vi "Write QueueMessageRef.vi"(8 "error in (no error)":errorcluster, 10 "QueueMessageRef":refnum<queue>, 11 "MicronGRPC in":refnum<class "MicronGRPC.lvclass">) -> (0 "error out":errorcluster, 3 "MicronGRPC out":refnum<class "MicronGRPC.lvclass">)   [LabVIEW 2019, in "MicronGRPCGeneratedServer.lvlib" / "MicronGRPC.lvclass"]
uses:
  MicronGRPC.lvclass
  Base/Server/Message/MessageBase.lvclass
  MicronGRPC.lvclass/MicronGRPC.ctl
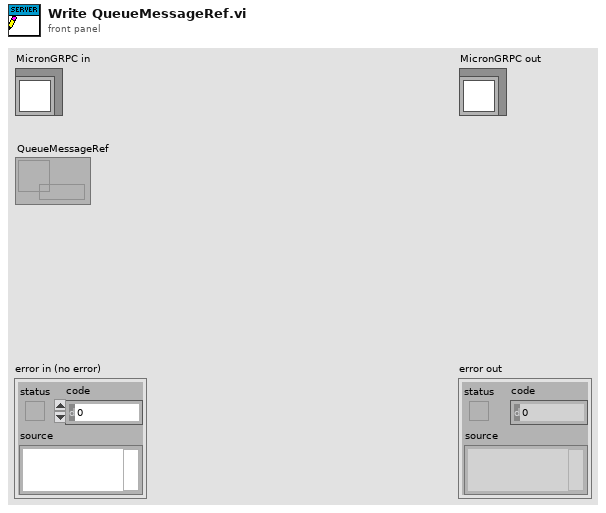
[diagram p1: front panel]
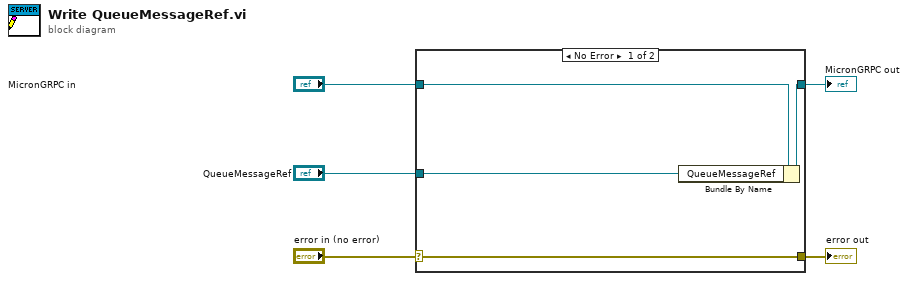
[diagram p0: block diagram]
diagram:
  n1 = case shown="No Error" "error in (no error)" {
    selector: "error in (no error)" -> [w9 w10]
    tunnel: [w9 w10] -> w4
    tunnel: [w7 w11] -> w2
    tunnel: "MicronGRPC in" -> [w8 w11]
    tunnel: "QueueMessageRef" -> [w6 _]
    frame No Error {
      n2 = Bundle By Name(cluster=w8, "QueueMessageRef"=w6) -> (w7:refnum<class "MicronGRPC.lvclass">)
    }
    frame Error {
    }
  }
  "error out" <- w4
  "MicronGRPC out" <- w2
